vi "Configure Output State.vi"(7 "Enable Output (T: Enable)":bool=TRUE, 8 "error in (no error)":errorcluster, 10 "Channel (0: 30V Channel)":T1 caption="Channel (0: +6V)" items=["30V/3A Channel", "30V/3A Channel", "5V/3A Channel"], 11 "VISA resource name":refnum<visa-resource-name>) -> (0 "error out":errorcluster, 3 "VISA resource name out":refnum<visa-resource-name>)   [LabVIEW 2020, in "Library Instrument & Equipement.lvlib" / "Library Power_Supply.lvlib" / "RIGOL DP800 Series.lvlib"]
doc: "Configures output voltage level, channel, and enables or disables the output of the power supply."
uses:
  RIGOL DP800 Series.lvlib
  Channels.ctl
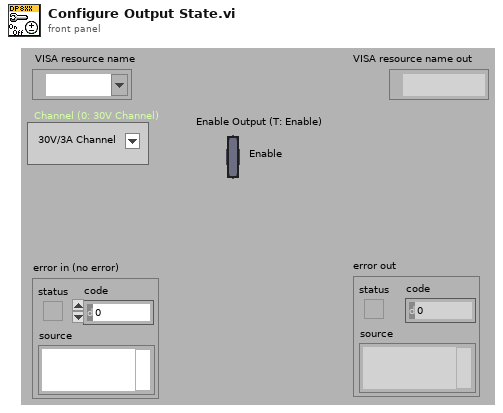
[diagram p1: front panel]
types:
  T1 = typedef "Library Instrument & Equipement.lvlib/Library Power_Supply.lvlib/RIGOL DP800 Series.lvlib/Channels.ctl" = i32
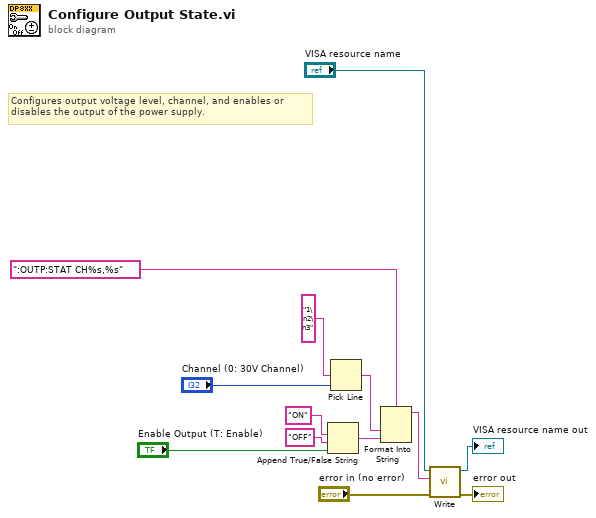
[diagram p0: block diagram]
diagram:
  # "Configures output voltage level, channel, and enables or \ndisables the output of the power supply."
  n1 = Append True/False String(1:"Enable Output (T: Enable)", 2:"OFF", 3:"ON") -> (0:w9:string)  [unwired: 1 out]
  n2 = Pick Line(multi-line string="1\n2\n3", line index="Channel (0: 30V Channel)") -> (output string=w7:string)  [unwired: 1 out]
  n3 = Format Into String(format string=":OUTP:STAT CH%s,%s", w7, w9) -> (resulting string=w1:string)  [unwired: 2 in, 1 out]
  n4 = call "Write.vi"("error in (no error)"="error in (no error)", "Write Buffer (\"\")"=w1, "VISA resource name"="VISA resource name") -> ("error out"=→"error out":errorcluster, "VISA resource name out"=→"VISA resource name out":refnum<visa-resource-name>)  [unwired: 7 in]
